vi "Full Adder From Half Adder.vi"() -> ()   [LabVIEW 2016]
panel:
  out "Carry":bool
  out "Sum":bool
  in  "C":bool
  in  "B":bool
  in  "A":bool
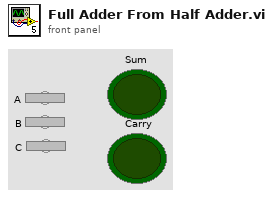
[diagram p1: front panel]
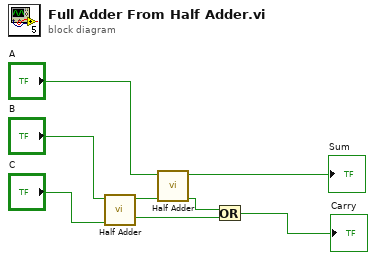
[diagram p0: block diagram]
diagram:
  n1 = call "Half Adder.vi"("B"="C", "A"="B") -> ("Carry"=w6:bool, "Sum"=w7:bool)  [unwired: 8 in]
  n2 = call "Half Adder.vi"("B"=w7, "A"="A") -> ("Carry"=w8:bool, "Sum"=→"Sum":bool)  [unwired: 8 in]
  n3 = Or(x=w8, y=w6) -> (x .or. y?=→"Carry":bool)
